vi "Solve2.vi"(8 "Error In":errorcluster, 11 "object in":refnum<class "2021_11.lvclass">) -> (0 "Error Out":errorcluster, 2 "Result":u64, 3 "object out":refnum<class "2021_11.lvclass">)   [LabVIEW 2020, in "2021_11.lvclass"]
uses:
  2021_11.lvclass
  2021_11.lvclass/2021_11.ctl
  6ae27fe5-da54-49ac-8b7e-7ebc6bf6ffa7.vi
  6ae27fe5-da54-49ac-8b7e-7ebc6bf6ffa7.vi/be6f088c-3e4b-4523-ad48-2cdc85bad38a.vi
  6ae27fe5-da54-49ac-8b7e-7ebc6bf6ffa7.vi/f202eadf-433e-4cdb-b986-b2351ce8d73c.vi
  6ae27fe5-da54-49ac-8b7e-7ebc6bf6ffa7.vi/094751bc-bcf2-4346-afae-53942128b536.vi
  6ae27fe5-da54-49ac-8b7e-7ebc6bf6ffa7.vi/06ee343e-764f-4086-89d5-f578778d243c.vi
panel:
  out "Round":i32
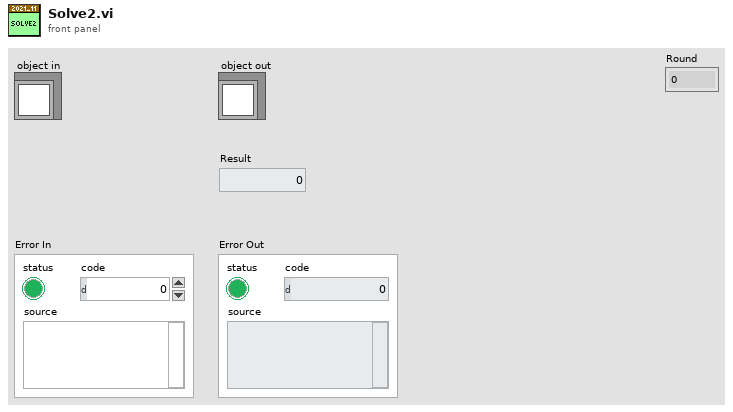
[diagram p1: front panel]
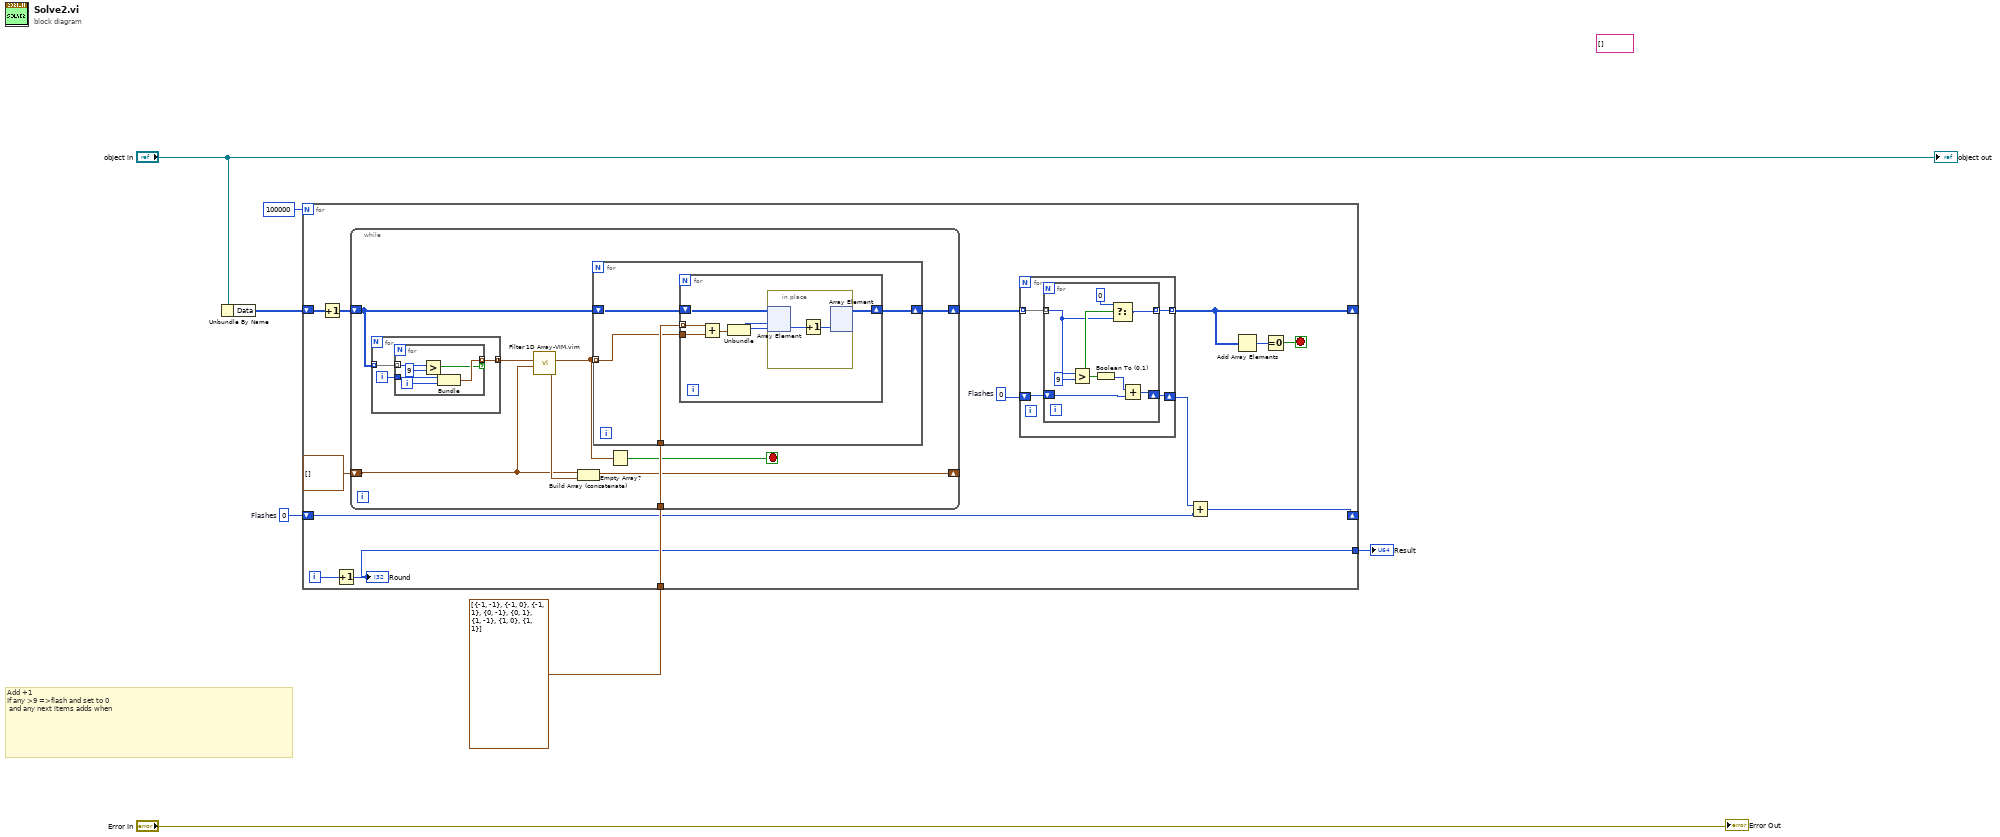
[diagram p0: block diagram]
diagram:
  w3 = 0  # Flashes
  (unwired) string[] [] ("LinesOfCode")
  # "Add +1\nIf any >9 =>flash and set to 0\n and any next items adds when"
  n1 = Unbundle By Name("object in") -> ("Data"=w5:i32[][])
  n2 = for {
    N: 100000 -> [_]
    shift-right: [w11] -> _
    shift-left: w5 -> [w21]
    shift-right: [w13] -> _
    shift-left: w3 -> [w15]
    tunnel: cluster{i32, i32}[] [{-1, -1}, {-1, 0}, {-1, 1}, {0, -1}, {0, 1}, {1, -1}, {1, 0}, {1, 1}] -> [w18]
    tunnel: [w8] -> w1
    i -> [w20]
    stop <- w9 stop-if-true
    w17 = 0  # Flashes
    n3 = Increment(x=w21) -> (x+1=w19:i32[][])
    n4 = Increment(x=w20) -> (x+1=w8:i32)
    "Round" <- w8
    n5 = while {
      tunnel: w18 -> [w28]
      shift-right: [w27] -> w16
      shift-left: w19 -> [w29]
      shift-right: [w24] -> _
      shift-left: cluster{i32, i32}[] [] -> [w22]
      stop <- w26 stop-if-true
      n6 = for {
        tunnel: w29 -> [w45] mode=indexing
        tunnel: [w43] -> w23 mode=concatenating
        i -> [w44]
        n7 = for {
          tunnel: w45 -> [w51] mode=indexing
          tunnel: w44 -> [w49]
          tunnel: [w47] -> w43 mode=indexing if=w46
          i -> [w48]
          n8 = Greater?(x=w51, y=9) -> (0:w46:bool)
          n9 = Bundle(w49, w48) -> (w47:cluster{i32, i32})  [unwired: 1 in]
        }
      }
      n10 = call "Filter 1D Array-VIM.vim"("Item(s) to Filter"=w22, "Array"=w23) -> ("Filtered Array"=w25:cluster{i32, i32}[])  [unwired: 5 in, 1 out]
      n11 = Build Array (concatenate)(w22, w25) -> (w24:cluster{i32, i32}[])
      n12 = for {
        tunnel: w25 -> [w31] mode=indexing
        shift-right: [w30] -> w27
        shift-left: w29 -> [w33]
        tunnel: w28 -> [w32]
        n13 = for {
          shift-right: [w34] -> w30
          shift-left: w33 -> [w38]
          tunnel: w32 -> [w40] mode=indexing
          tunnel: w31 -> [w39]
          n14 = Add(x=w40, y=w39) -> (x+y=w37:cluster{i32, i32})
          n15 = Unbundle(w37) -> (w36:i32, w35:i32)
          n16 = in-place {
            n17 = in-place-array #1(w38, w36, w35) -> (w42:i32)
            n18 = Increment(x=w42) -> (x+1=w41:i32)
            n19 = in-place-array #1(w41) -> (w34:i32[][])  [unwired: 2 out]
          }
        }
      }
      n20 = Empty Array?(array=w25) -> (empty?=w26:bool)
    }
    n21 = for {
      shift-right: [w53] -> w14
      shift-left: w17 -> [w55]
      tunnel: w16 -> [w54] mode=indexing
      tunnel: [w52] -> w11 mode=indexing
      n22 = for {
        shift-right: [w60] -> w53
        shift-left: w55 -> [w62]
        tunnel: w54 -> [w57] mode=indexing
        tunnel: [w56] -> w52 mode=indexing
        n23 = Greater?(x=w57, y=9) -> (0:w59:bool)
        n24 = Boolean To (0,1)(Boolean=w59) -> (0, 1=w61:i16)
        n25 = Select(t=0 ("y"), s=w59, f=w57) -> (s? t:f=w56:i32)
        n26 = Add(x=w61, y=w62) -> (x+y=w60:i32)
      }
    }
    n27 = Add(x=w14, y=w15) -> (x+y=w13:i32)
    n28 = Add Array Elements(numeric array=w11) -> (sum=w10:i32)
    n29 = Equal To 0?(x=w10) -> (x = 0?=w9:bool)
  }
  "Result" <- w1
  "Error Out" <- "Error In"
  "object out" <- "object in"
